vi "AddNewValue.vi"(6 "Data Cluster":T1, 8 "error IO":errorcluster, 9 "DataType and Value":cluster{"Type":string, "Value":variant}, 11 "Data":T2) -> (0 "error IO Out":errorcluster, 2 "DataType and Value Out":cluster{"Type":string, "Value":variant}, 3 "JSON Text Out":string)   [LabVIEW 2017]
uses:
  Ctrl/Property.ctl
  Ctrl/PhysicalChannel.ctl
  Ctrl/Bitfield.ctl
  Ctrl/Register.ctl
  Ctrl/ScaleType.ctl
  Ctrl/Scale.ctl
  Ctrl/EnumValue.ctl
  Ctrl/Enum.ctl
  Ctrl/Caps.ctl
  Ctrl/Data.ctl
  Ctrl/UserInput.ctl
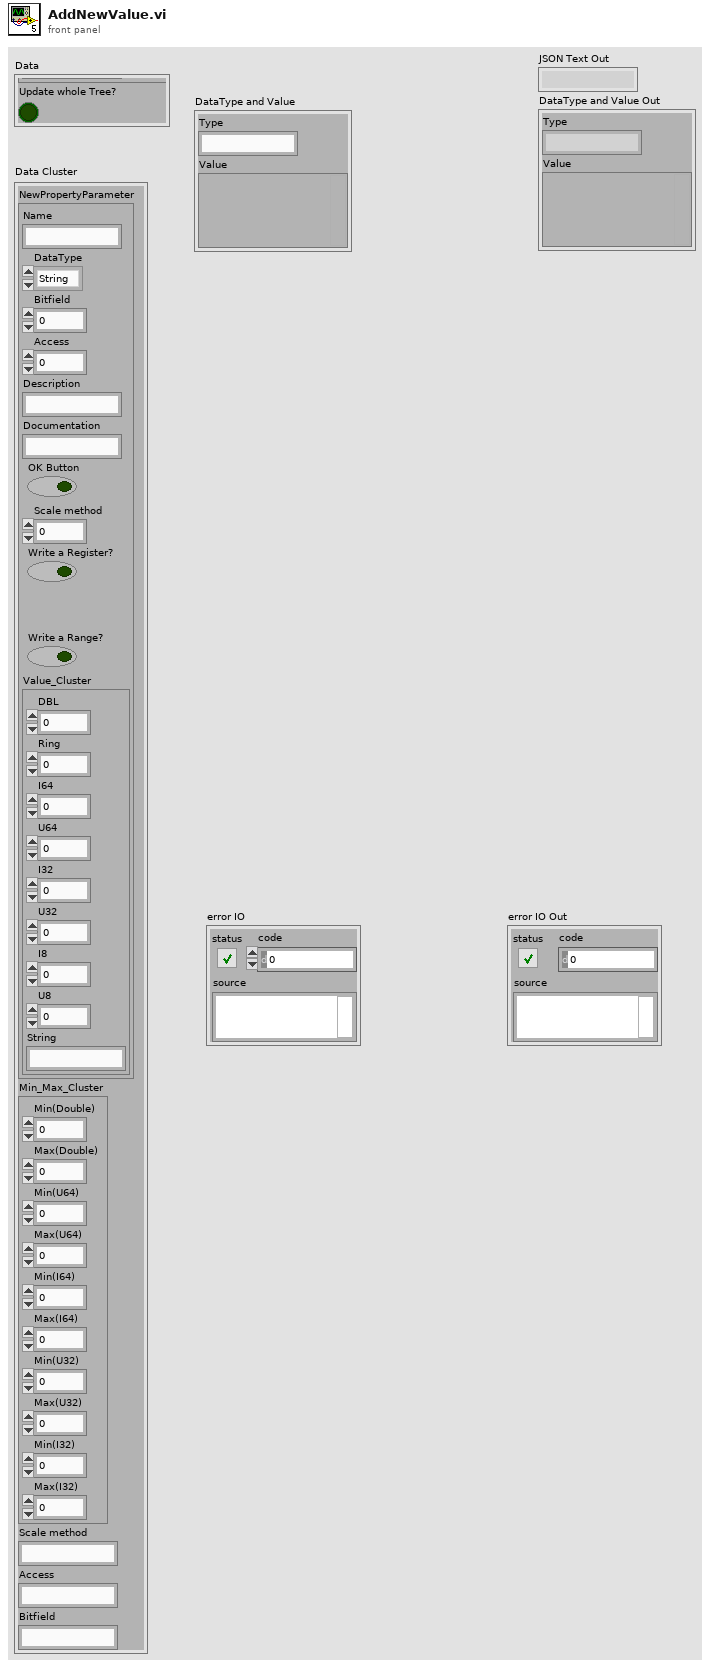
[diagram p1: front panel]
types:
  T1 = typedef "UserInput.ctl" = cluster{"NewPropertyParameter":cluster{"Name":string, "DataType":enum16{"String", "Double", "U64", "I64", "U32", "I32", "Bool"}, "Bitfield":u16, "Access":u16, "Description":string, "Documentation":string, "OK Button":bool, "Scale method":u16, "Write a Register?":bool, "Write a Range?":bool, "Value_Cluster":cluster{"DBL":dbl, "Ring":u16, "I64":i64, "U64":u64, "I32":i32, "U32":u32, "I8":i8, "U8":u8, "String":string}}, "Min_Max_Cluster":cluster{"Min(Double)":dbl, "Max(Double)":dbl, "Min(U64)":u64, "Max(U64)":u64, "Min(I64)":i64, "Max(I64)":i64, "Min(U32)":u32, "Max(U32)":u32, "Min(I32)":i32, "Max(I32)":i32}, "Scale method":string, "Access":string, "Bitfield":string}
  T2 = typedef "Data.ctl" = cluster{"Ref Cluster":cluster{"String":refnum<vi>, "U8":refnum<vi>, "I8":refnum<vi>, "U32":refnum<vi>, "I32":refnum<vi>, "U64":refnum<vi>, "I64":refnum<vi>, "Ring":refnum<vi>, "DBL":refnum<vi>, "Add":refnum<vi>, "Remove":refnum<vi>, "Property tree":refnum<vi>}, "JSON Text":string, "Original JSON Text":string, "Caps":T3, "SLSC Output Tree":cluster{"Left Cell String":string, "Child Text":string[], "Child Tag":string, "Item Indent":i32, "Child Only?":bool, "Glyph Index":i32, "offline value":variant}[], "Ref Index and Control Type":cluster{"index":i32, "Datatype":string}, "Selected Type and name":cluster{"Selected Type":enum16{"Property", "Physical Channel", "Other"}, "Selected Property Name":string}, "Update whole Tree?":bool}
  T3 = typedef "Caps.ctl" = cluster{"properties":T4[], "physical channels":T5[], "registers":T6[], "scales":T8[], "enums":T10[], "productName":string}
  T4 = typedef "Property.ctl" = cluster{"name":string, "bitfield":string, "value":variant, "dataType":string, "min":variant, "max":variant, "scale":string, "access":string}
  T5 = typedef "PhysicalChannel.ctl" = cluster{"name":string, "properties":T4[]}
  T6 = typedef "Register.ctl" = cluster{"name":string, "address":i32, "size":i32, "bitfields":T7[], "initialValue":variant, "connectedProperties":string[]}
  T7 = typedef "Bitfield.ctl" = cluster{"name":string, "offset":i32, "size":i32, "signed":bool}
  T8 = typedef "Scale.ctl" = cluster{"name":string, "type":T9, "params":variant}
  T9 = typedef "ScaleType.ctl" = enum16{"NoScale", "Table", "Polynomial", "Linear"}
  T10 = typedef "Enum.ctl" = cluster{"name":string, "values":T11[]}
  T11 = typedef "EnumValue.ctl" = cluster{"name":string, "value":i32}
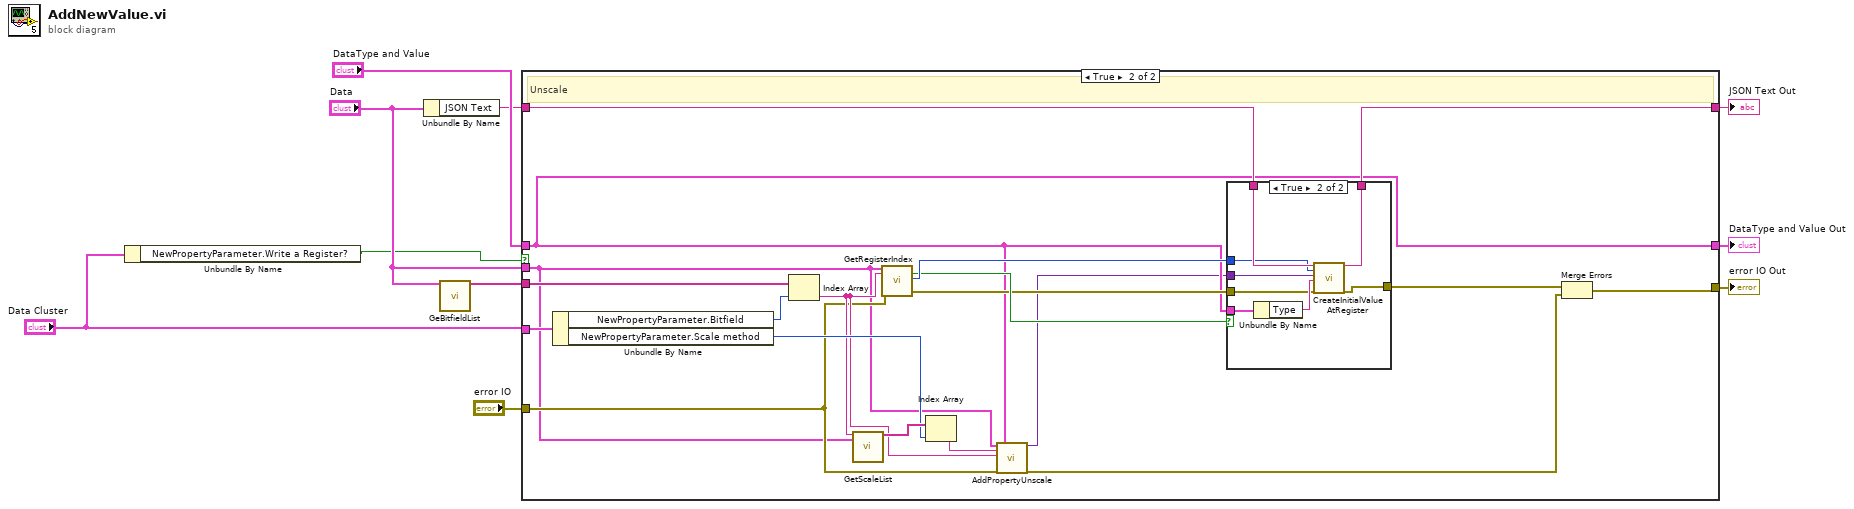
[diagram p0: block diagram]
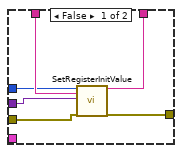
[diagram p3: hidden frame]
diagram:
  n1 = Unbundle By Name("Data Cluster") -> ("NewPropertyParameter.Write a Register?"=w1:bool)
  n2 = Unbundle By Name("Data") -> ("JSON Text"=w7:string)
  n3 = call "GeBitfieldList.vi"("Data"="Data") -> ("Array"=w10:string[])  [unwired: 18 in]
  n4 = case shown="True" w1 {
    tunnel: "DataType and Value" -> [w11 w19]
    tunnel: w7 -> [w13 w32]
    tunnel: [w13 w31] -> w5
    tunnel: [w12 w16] -> w3
    tunnel: "error IO" -> [w12 w17]
    tunnel: [w11 w19] -> w4
    tunnel: "Data Cluster" -> [_ w29]
    tunnel: w10 -> [_ w28]
    tunnel: "Data" -> [_ w14]
    frame False {
    }
    frame True {
      # "Unscale"
      n5 = Unbundle By Name(w29) -> ("NewPropertyParameter.Bitfield"=w27:u16, "NewPropertyParameter.Scale method"=w22:u16)
      n6 = Index Array(array=w28, index=w27) -> (element=w20:string)
      n7 = call "GetScaleList.vi"("Bitfield in"=w20, "Data in"=w14) -> ("output array"=w23:string[])  [unwired: 17 in]
      n8 = call "GetRegisterIndex.vi"("Data"=w14, "Bitfield"=w20, "error in (no error)"=w17) -> ("Empty?"=w25:bool, "Index"=w26:i32, "error out"=w24:errorcluster)  [unwired: 13 in, 1 out]
      n9 = Index Array(array=w23, index=w22) -> (element=w21:string)
      n10 = call "AddPropertyUnscale.vi"("Data"=w14, "Scale method"=w21, "Bitfield"=w20, "error in"=w17, "Type&Value"=w19) -> ("Variant"=w18:variant, "error out"=w15:errorcluster)  [unwired: 13 in]
      n11 = case shown="True" w25 {
        tunnel: w32 -> [w38 w46]
        tunnel: [w37 w45] -> w31
        tunnel: [w36 w41] -> w30
        tunnel: w26 -> [w35 w44]
        tunnel: w19 -> [_ w43]
        tunnel: w18 -> [w34 w40]
        tunnel: w24 -> [w33 w39]
        frame False {
          n12 = call "SetRegisterInitValue.vi"("Index"=w35, "JSON"=w38, "Variant"=w34, "error in (no error)"=w33) -> ("<JSON>"=w37:string, "error out"=w36:errorcluster)  [unwired: 12 in, 2 out]
        }
        frame True {
          n13 = Unbundle By Name(w43) -> ("Type"=w42:string)
          n14 = call "CreateInitialValueAtRegister.vi"("JSON"=w46, "Register Index"=w44, "Value"=w40, "DataType"=w42, "error in (no error)"=w39) -> ("<JSON>"=w45:string, "error out"=w41:errorcluster)  [unwired: 13 in]
        }
      }
      n15 = Merge Errors(w30, w15) -> (w16:errorcluster)
    }
  }
  "JSON Text Out" <- w5
  "DataType and Value Out" <- w4
  "error IO Out" <- w3
